vi "ShooterIntakeWheelControl.vi"(0 "Constants":T1={"motorConstants"={"leftDriveMotor"=0, "rightDriveMotor"=0, "climberWinch"=enum."PWM 0", "shooterTopFlyWheel"=enum."PWM 0", "shooterBottomFlyWheel"=enum."PWM 0", "climberExtender"=enum."PWM 0", "shooterIntakeWheel"=0, "Front Arm Motor"=0}, "arduinoInputChannel"={"armAngleUp"=0, "intakeWheelSpinIn"=0, "winchUp"=0, "extenderUp"=0, "AimingAuto"=0, "extenderDown"=0, "FrontArmAxis"=0, "shooter up/down"=0}, "driveConstants"={"firstIntervalPercent"=0.0, "secondIntervalPercent"=0.0, "thirdIntervalPercent"=0.0}, "cRioInputChanels"={"photoEye"=0, "limitExtender"=0}, "pneumaticsChannels"={"angleSolenoid"=enum."Solenoid 0", "shooterAnglerPneumaticForward"=enum."Solenoid 0", "shooterAnglerPneumaticReverse"=enum."Solenoid 0", "Pneumatics Control Module"=1, "Ball Stopper Forward"=enum."Solenoid 0", "Ball Stopper Reverse"=enum."Solenoid 0"}, "flyWheelConstants"={"manualTopWheel"=0.0, "manualBottomWheel"=0.0, "autoFuncConst1"=0.0, "autoFuncConst2"=0.0, "autoFuncConst3"=0.0, "autoFuncConst4"=0.0, "Array"=[]}}, 1 "leonardoJoystick":bool[](array[boolean]), 2 "driverJoystickLeft":bool[](array[boolean]), 3 "driverJoystickRight":bool[](array[boolean])) -> ()   [LabVIEW 2015]
doc: "logic for controling the intake wheel from up positions.\nchecks trigger buttons from left and right joystick to decide if we wanna fire"
uses:
  constants/constants.ctl
  <vilib>/Rock Robotics/SystemInterfaces/DIO/FPGA_DIOPWMChannel.ctl
  <vilib>/Rock Robotics/WPI/Solenoid/WPI_SolenoidChannel.ctl
panel:
  # "ShooterMotors"
  # "DriveMotors- CAN Bus"
  # "PWM"
  # "ClimberMotors"
  # "PWM"
  # "PWM"
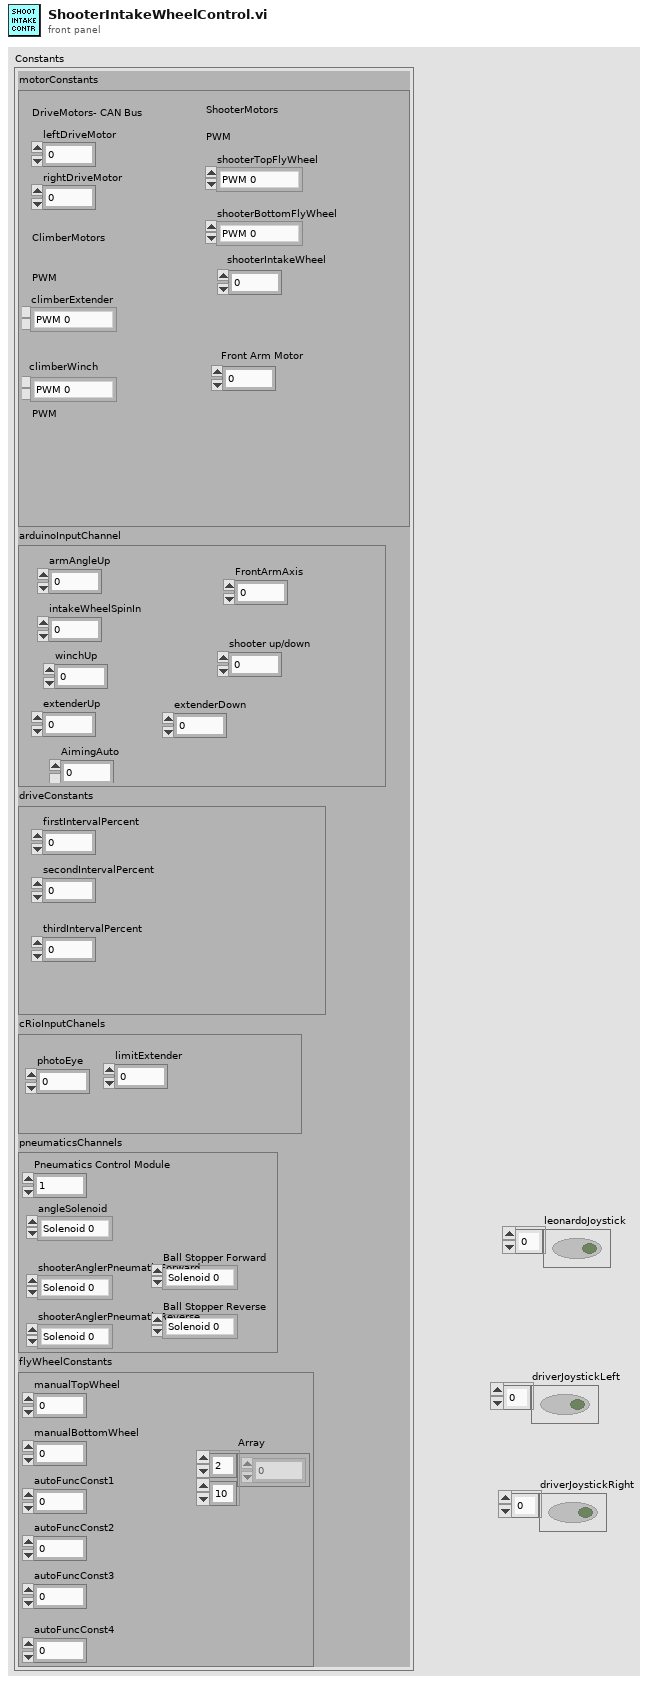
[diagram p1: front panel]
types:
  T1 = typedef "constants.ctl" = cluster{"motorConstants":cluster{"leftDriveMotor":u8, "rightDriveMotor":u8, "climberWinch":T2, "shooterTopFlyWheel":T2, "shooterBottomFlyWheel":T2, "climberExtender":T2, "shooterIntakeWheel":u8, "Front Arm Motor":u8}, "arduinoInputChannel":cluster{"armAngleUp":i32, "intakeWheelSpinIn":i32, "winchUp":i32, "extenderUp":i32, "AimingAuto":i32, "extenderDown":i32, "FrontArmAxis":i32, "shooter up/down":i32}, "driveConstants":cluster{"firstIntervalPercent":dbl, "secondIntervalPercent":dbl, "thirdIntervalPercent":dbl}, "cRioInputChanels":cluster{"photoEye":i32, "limitExtender":i32}, "pneumaticsChannels":cluster{"angleSolenoid":T3, "shooterAnglerPneumaticForward":T3, "shooterAnglerPneumaticReverse":T3, "Pneumatics Control Module":u8, "Ball Stopper Forward":T3, "Ball Stopper Reverse":T3}, "flyWheelConstants":cluster{"manualTopWheel":dbl, "manualBottomWheel":dbl, "autoFuncConst1":dbl, "autoFuncConst2":dbl, "autoFuncConst3":dbl, "autoFuncConst4":dbl, "Array":dbl[][]}}
  T2 = typedef "FPGA_DIOPWMChannel.ctl" = enum8{"PWM 0", "PWM 1", "PWM 2", "PWM 3", "PWM 4", "PWM 5", "PWM 6", "PWM 7", "PWM 8", "PWM 9", "PWM MXP 0", "PWM MXP 1", "PWM MXP 2", "PWM MXP 3", "PWM MXP 4", "PWM MXP 5", "PWM MXP 6", "PWM MXP 7", "PWM MXP 8", "PWM MXP 9", "Invalid"}
  T3 = typedef "WPI_SolenoidChannel.ctl" = enum8{"Solenoid 0", "Solenoid 1", "Solenoid 2", "Solenoid 3", "Solenoid 4", "Solenoid 5", "Solenoid 6", "Solenoid 7", "Invalid"}
  T4 = typedef "WPI_MotorControlDeviceRef.ctl" = cluster{"DeviceStatus":errorcluster, "Type":T5, "PWM":cluster{"PWM Channel":T2, "DeadBand":T6}, "CAN":cluster{"Device Number":u8, "Control Mode":T7, "Semaphore":T8, "Max Vout":dbl, "TalonSRX Control Mode":T9}, "Invert":bool}
  T5 = typedef "WPI_MotorControlType.ctl" = enum16{"PWM", "CAN", "CANTalonSRX"}
  T6 = typedef "WPI_PWMDeadband.ctl" = cluster{"Name":string, "maxPositivePwm":i32, "minPositivePwm":i32, "centerPwm":i32, "maxNegativePwm":i32, "minNegativePwm":i32, "angularRange":u16}
  T7 = typedef "WPI_CANJaguar_ControlMode.ctl" = enum8{"Percent VBus", "Current", "Speed", "Position", "Voltage"}
  T8 = typedef "Semaphore RefNum" = refnum<k1>
  T9 = typedef "WPI_CANTalonSRX_APIControlMode.ctl" = enum8{"Percent VBus", "Speed", "Position", "Slave", "Unchanged / Invalid", "Voltage Compensation", "Current", "Motion Profile"}
  T10 = typedef "WPI_CANTalonSRX_GlobalStatus.ctl" = cluster{"Applied Throttle":dbl, "Module Enabled":bool, "CAN Error":errorcluster, "Closed Loop Error":dbl, "Forward Limit Switch Closed":bool, "Reverse Limit Switch Closed":bool, "Sensor Position":dbl, "Sensor Velocity":dbl, "Current":dbl, "Sticky Fault - Over Temp":bool, "Sticky Fault - Under Voltage":bool, "Sticky Fault - Forward Limit":bool, "Sticky Fault - Reverse Limit":bool, "Sticky Fault - Forward Soft Limit":bool, "Sticky Fault - Reverse Soft Limit":bool, "Brake is Enabled":bool, "Encoder Position":dbl, "Encoder Velocity":dbl, "Encoder Index Count":dbl, "Encoder A Pin State":bool, "Encoder B Pin State":bool, "Encoder Index Pin State":bool, "Analog In":dbl, "Analog In Velocity":dbl, "Temperature (C)":dbl, "Battery Voltage":dbl, "Control 5 Is Supported":bool, "Current Profile Slot Select":dbl, "Pos Div 8":bool, "Vel Div 4":bool, "Pulse Width Position":i32, "Pulse Width Velocity":i32, "Pulse Width Rise To Rise (us)":i32, "Pulse Width Rise To Fall (us)":i32, "Mot Prof Active Is Under Run":bool, "Mot Prof Active Has Under Run":bool, "Mot Prof Active Is Last":bool, "Mot Prof Active Velocity Only":bool, "Mot Prof Active Is Valid":bool, "Mot Prof Buffer Is Full":bool, "Mot Prof Active Profile Slot Select":i32, "Mot Prof NextID":i32, "Mot Prof Count":i32, "Mot Prof Active Velocity":dbl, "Mot Prof Active Position":dbl, "Mot Prof Output Enable":i32}
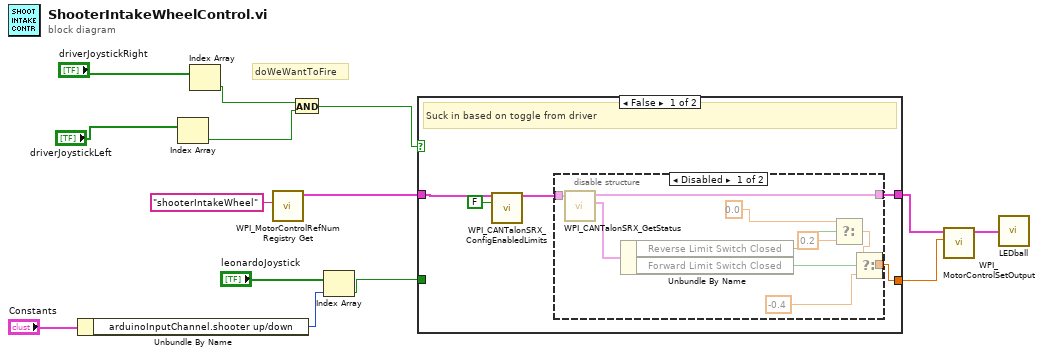
[diagram p0: block diagram]
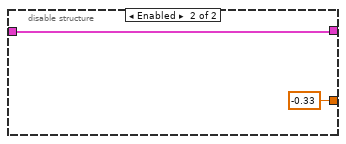
[diagram p2: hidden frame]
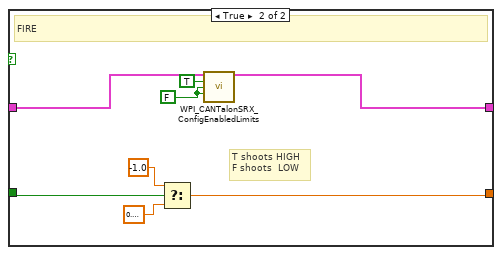
[diagram p3: hidden frame]
diagram:
  # "doWeWantToFire"
  n1 = Unbundle By Name("Constants") -> ("arduinoInputChannel.shooter up/down"=w13:i32)
  n2 = Index Array(array="driverJoystickLeft") -> (element=w7:bool)  [unwired: 1 in]
  n3 = Index Array(array="driverJoystickRight") -> (element=w8:bool)  [unwired: 1 in]
  n4 = call <vilib>:"WPI_MotorControlRefNum Registry Get.vi"("refnum name"="shooterIntakeWheel") -> ("MotorControlDevRef"=w3:T4)  [unwired: 9 in, 1 out]
  n5 = And(x=w8, y=w7) -> (x .and. y?=w6:bool)
  n6 = Index Array(array="leonardoJoystick", index=w13) -> (element=w5:bool)
  n7 = case shown="False" w6 {
    tunnel: w5 -> [_ w39]
    tunnel: [w15 w36] -> w4
    tunnel: w3 -> [w18 w35]
    tunnel: [w16 w33] -> w1
    frame False {
      # "Suck in based on toggle from driver"
      n8 = call <vilib>:"WPI_CANTalonSRX_ConfigEnabledLimits.vi"("CAN Talon SRX Ref"=w18, "Override Limit Switches"=FALSE) -> ("CAN Talon SRX Ref"=w17:T4)  [unwired: 12 in, 1 out]
      n9 = disable-structure shown="Disabled" {
        disable-tunnel: w17 -> [w29 w31]
        disable-tunnel: [w28 w31] -> w16
        disable-tunnel: [w26 -0.33 ("f")] -> w15
        frame Disabled {
          n10 = call <vilib>:"WPI_CANTalonSRX_GetStatus.vi"("CAN Talon SRX Ref"=w29) -> ("Talon SRX Status"=w27:T10, "CAN Talon SRX Ref"=w28:T4)  [unwired: 8 in, 1 out]
          n11 = Unbundle By Name(w27) -> ("Reverse Limit Switch Closed"=w22:bool, "Forward Limit Switch Closed"=w25:bool)
          n12 = Select(t=0.0, s=w22, f=0.2) -> (s? t:f=w21:dbl)
          n13 = Select(t=w21, s=w25, f=-0.4) -> (s? t:f=w26:dbl)
        }
        frame Enabled {
        }
      }
    }
    frame True {
      w32 = FALSE ("Forward Limit Switch Enable")
      # "T shoots HIGH\nF shoots  LOW"
      # "FIRE"
      n14 = Select(t=-1.0, s=w39, f=0.7999999999999999) -> (s? t:f=w36:dbl)
      n15 = call <vilib>:"WPI_CANTalonSRX_ConfigEnabledLimits.vi"("CAN Talon SRX Ref"=w35, "Override Limit Switches"=TRUE, "Forward Limit Switch Enable"=w32, "Reverse Limit Switch Enable"=w32) -> ("CAN Talon SRX Ref"=w33:T4)  [unwired: 10 in, 1 out]
    }
  }
  n16 = call <vilib>:"WPI_MotorControlSetOutput.vi"("Output"=w4, "MotorControlDevRef"=w1) -> ("MotorControlDevRef"=w2:T4)  [unwired: 7 in, 2 out]
  n17 = call "LEDball.vi"("MotorControlDevRef"=w2) -> ()
